vi "Write Needed Number.vi"(8 "error in (no error)":errorcluster, 10 "Needed Number":u32, 11 "AbstractCollector in":refnum<class "AbstractCollector.lvclass">) -> (0 "error out":errorcluster, 3 "AbstractCollector out":refnum<class "AbstractCollector.lvclass">)   [LabVIEW 2014, in "AbstractCollector.lvclass"]
uses:
  AbstractCollector.lvclass
  AbstractCollector.lvclass/AbstractCollector.ctl
  Interfaces/Observable Actor/Observable Actor.lvclass
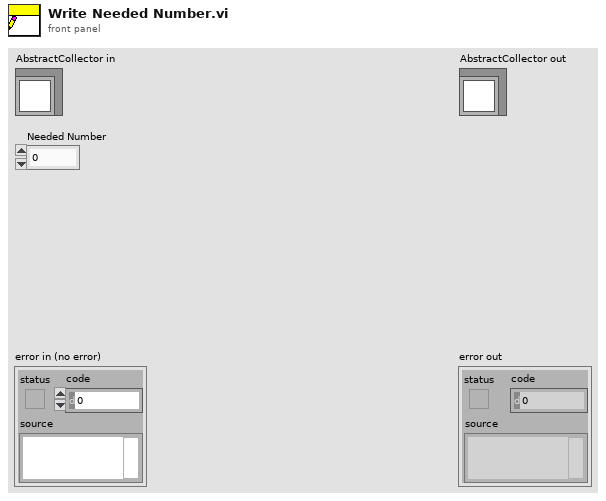
[diagram p1: front panel]
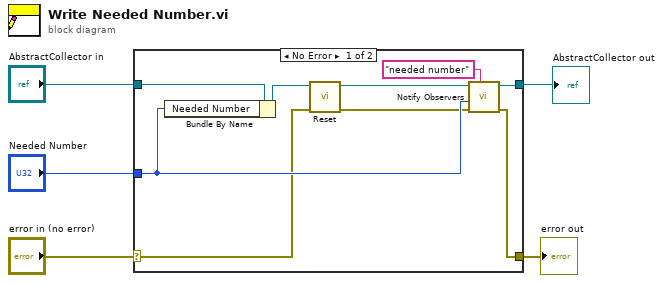
[diagram p0: block diagram]
diagram:
  n1 = case shown="No Error" "error in (no error)" {
    selector: "error in (no error)" -> [w8 w15]
    tunnel: [w12 w15] -> w4
    tunnel: [w13 w16] -> w2
    tunnel: "AbstractCollector in" -> [w14 w16]
    tunnel: "Needed Number" -> [w11 _]
    frame No Error {
      n2 = Bundle By Name(cluster=w14, "Needed Number"=w11) -> (w9:refnum<class "AbstractCollector.lvclass">)
      n3 = call-dynamic "Reset.vi"("error in (no error)"=w8, "AbstractCollector in"=w9) -> ("error out"=w7:errorcluster, "AbstractCollector out"=w6:refnum<class "AbstractCollector.lvclass">)  [unwired: 8 in]
      n4 = call "Notify Observers.vi"("name"="needed number", "error in (no error)"=w7, "value"=w11, "Observable Actor in"=w6) -> ("error out"=w12:errorcluster, "Observable Actor out"=w13:refnum<class "AbstractCollector.lvclass">)  [unwired: 6 in]
    }
    frame Error {
    }
  }
  "error out" <- w4
  "AbstractCollector out" <- w2
